vi "Close.vi"(8 "error in":errorcluster, 11 "DAQmx Base CFG in":refnum<class "DAQmx Base CFG.lvclass">) -> (0 "error out":errorcluster, 3 "DAQmx Base CFG out":refnum<class "DAQmx Base CFG.lvclass">)   [LabVIEW 2023, in "DAQmx Base CFG.lvclass"]
uses:
  DAQmx Base CFG.lvclass
  DAQmx Base CFG.lvclass/DAQmx Base CFG.ctl
  Configurations/CFG JSON/CFG JSON.lvclass
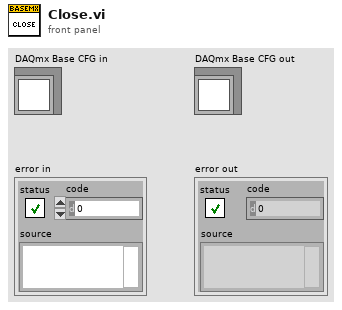
[diagram p1: front panel]
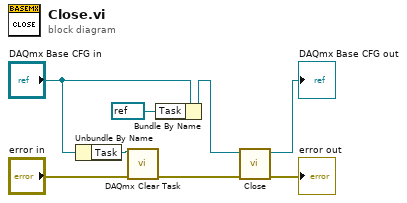
[diagram p0: block diagram]
diagram:
  n1 = Unbundle By Name("DAQmx Base CFG in") -> ("Task"=w1:refnum<k21>)
  n2 = call <vilib>:"DAQmx Clear Task.vi"("task in"=w1, "error in"="error in") -> ("error out"=w5:errorcluster)  [unwired: 13 in]
  n3 = Bundle By Name(cluster="DAQmx Base CFG in", "Task"=refnum<k21> refnum) -> (w3:refnum<class "DAQmx Base CFG.lvclass">)
  n4 = call-parent "Close.vi"("error in"=w5, "CFG Base in"=w3) -> ("error out"=→"error out":errorcluster, "CFG Base out"=→"DAQmx Base CFG out":refnum<class "DAQmx Base CFG.lvclass">)  [unwired: 8 in]
